vi "Shutdown.vi"(8 "error in (no error)":errorcluster, 11 "Type Converter in":refnum<class "Default Buffer Converter.lvclass">) -> (0 "error out":errorcluster, 3 "Type Converter out":refnum<class "Default Buffer Converter.lvclass">)   [LabVIEW 2017, in "DSF Core.lvlib" / "Default Buffer Converter.lvclass"]
uses:
  Default Buffer Converter.lvclass
  Default Buffer Converter.lvclass/Default Buffer Converter.ctl
  Conversion.ctl
  Conversion Block.ctl
  Typedefs/DSF Data Type.ctl
  DSF Core.lvlib
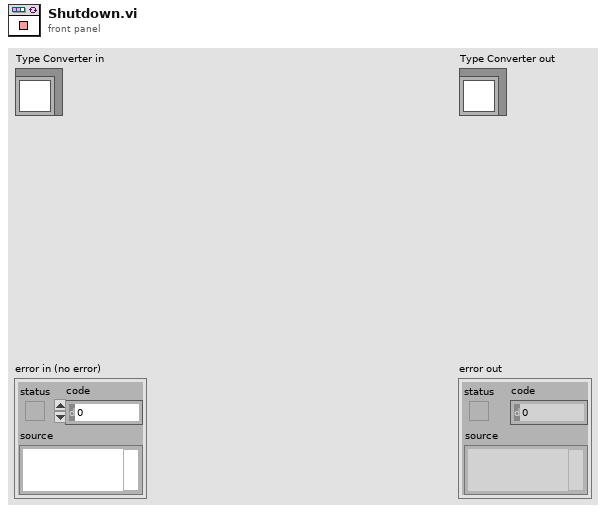
[diagram p1: front panel]
types:
  T1 = typedef "DSF Core.lvlib/Default Buffer Converter.lvclass/Conversion.ctl" = cluster{"conversion blocks":T2[]}
  T2 = typedef "DSF Core.lvlib/Default Buffer Converter.lvclass/Conversion Block.ctl" = cluster{"engine offset":u64, "engine data type":T3, "string offset":u64, "string data type":T3, "engine byte order":enum16{"big-endian, network order", "native, host order", "little-endian"}, "string byte order":enum16{"big-endian, network order", "native, host order", "little-endian"}, "count":u64}
  T3 = typedef "DSF Core.lvlib/DSF Data Type.ctl" = enum8{"Bool", "SGL", "DBL", "I8", "I16", "I32", "I64", "U8", "U16", "U32", "U64"}
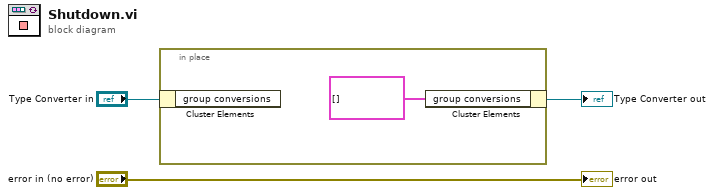
[diagram p0: block diagram]
diagram:
  n1 = in-place {
    n2 = in-place-cluster #1("Type Converter in") -> ()  [unwired: 1 out]
    n3 = in-place-cluster #1("group conversions"=T1[] [] ("conversions")) -> (→"Type Converter out":refnum<class "Default Buffer Converter.lvclass">)
  }
  "error out" <- "error in (no error)"
